vi "Self.vi"(9 "Priority?":bool, 10 "Msg Strategy":refnum<class "Msg Strategy.lvclass">, 11 "Base jettl in":refnum<class "Base jettl.lvclass">) -> (3 "Base jettl out":refnum<class "Base jettl.lvclass">)   [LabVIEW 2021, in "jettl.lvlib" / "Base jettl.lvclass"]
uses:
  Base jettl.lvclass
  Msg Strategy/Msg Strategy.lvclass
  Base jettl.lvclass/Base jettl.ctl
  Addresses Strategy/Addresses Strategy/Addresses Strategy.lvclass
  Sender/Sender.lvlib
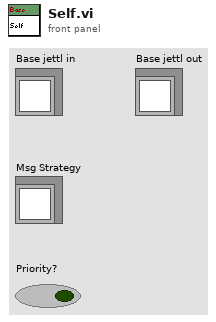
[diagram p1: front panel]
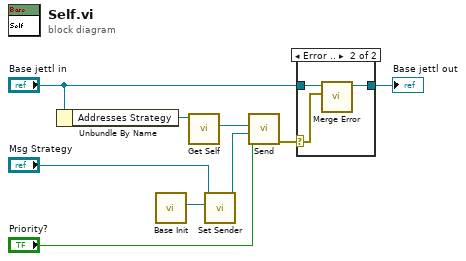
[diagram p0: block diagram]
diagram:
  n1 = Unbundle By Name("Base jettl in") -> ("Addresses Strategy"=w9:refnum<class "Addresses Strategy.lvclass">)
  n2 = call "Base Init.vi"() -> ("Sender"=w1:refnum<class "Sender.lvclass">)  [unwired: 11 in]
  n3 = call-dynamic "Get Self.vi"("Addresses Strategy in"=w9) -> ("Self"=w6:refnum<user-event>)  [unwired: 10 in]
  n4 = call-dynamic "Set Sender.vi"("Sender"=w1, "Msg Strategy in"="Msg Strategy") -> ("Msg Strategy out"=w2:refnum<class "Msg Strategy.lvclass">)  [unwired: 9 in]
  n5 = call "Send.vi"("Priority?"="Priority?", "Msg Strategy"=w2, "Msg Event"=w6) -> ("error out"=w4:errorcluster)  [unwired: 8 in]
  n6 = case shown="Error .." w4 {
    selector: w4 -> [_ w11]
    tunnel: [w10 w13] -> w7
    tunnel: "Base jettl in" -> [w10 w12]
    frame No Error {
    }
    frame Error {
      n7 = call-dynamic "Merge Error.vi"("Error"=w11, "Base jettl in"=w12) -> ("Base jettl out"=w13:refnum<class "Base jettl.lvclass">)  [unwired: 9 in]
    }
  }
  "Base jettl out" <- w7
